vi "Test.vi"() -> ()   [LabVIEW 2022 SP3, in "ZKTimingControl.lvlib" / "TimingControl.lvclass"]
uses:
  TimingControl.lvclass
panel:
  in  "仪器状态":bool
  out "数据":cluster{"启动":bool, "控制命令":T1, "测量参数":T2}={"启动"=FALSE, "控制命令"=enum."加标回收（启动采配水）", "测量参数"={"氨氮"=TRUE, "总磷"=TRUE, "总氮"=TRUE, "CODMn"=TRUE, "CODCr"=FALSE, "氟化物"=FALSE, "挥发酚"=FALSE}}
  in  "布尔":bool
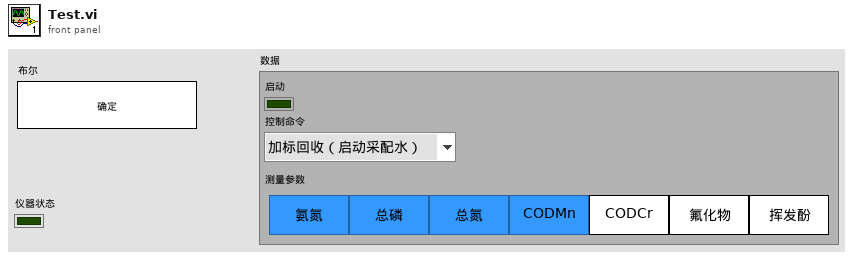
[diagram p1: front panel]
types:
  T1 = typedef "ZKTimingControl.lvlib/TimingControl.lvclass/国标控制命令.ctl" = enum16{"加标回收（启动采配水）", "加标回收（不启动采配水）", "水样测试（启动采配水）", "水样测试（不启动采配水）", "平行样测试（启动采配水）", "平行样测试（不启动采配水）", "集成干预测试"}
  T2 = typedef "ZKTimingControl.lvlib/TimingControl.lvclass/测量参数.ctl" = cluster{"氨氮":bool, "总磷":bool, "总氮":bool, "CODMn":bool, "CODCr":bool, "氟化物":bool, "挥发酚":bool}
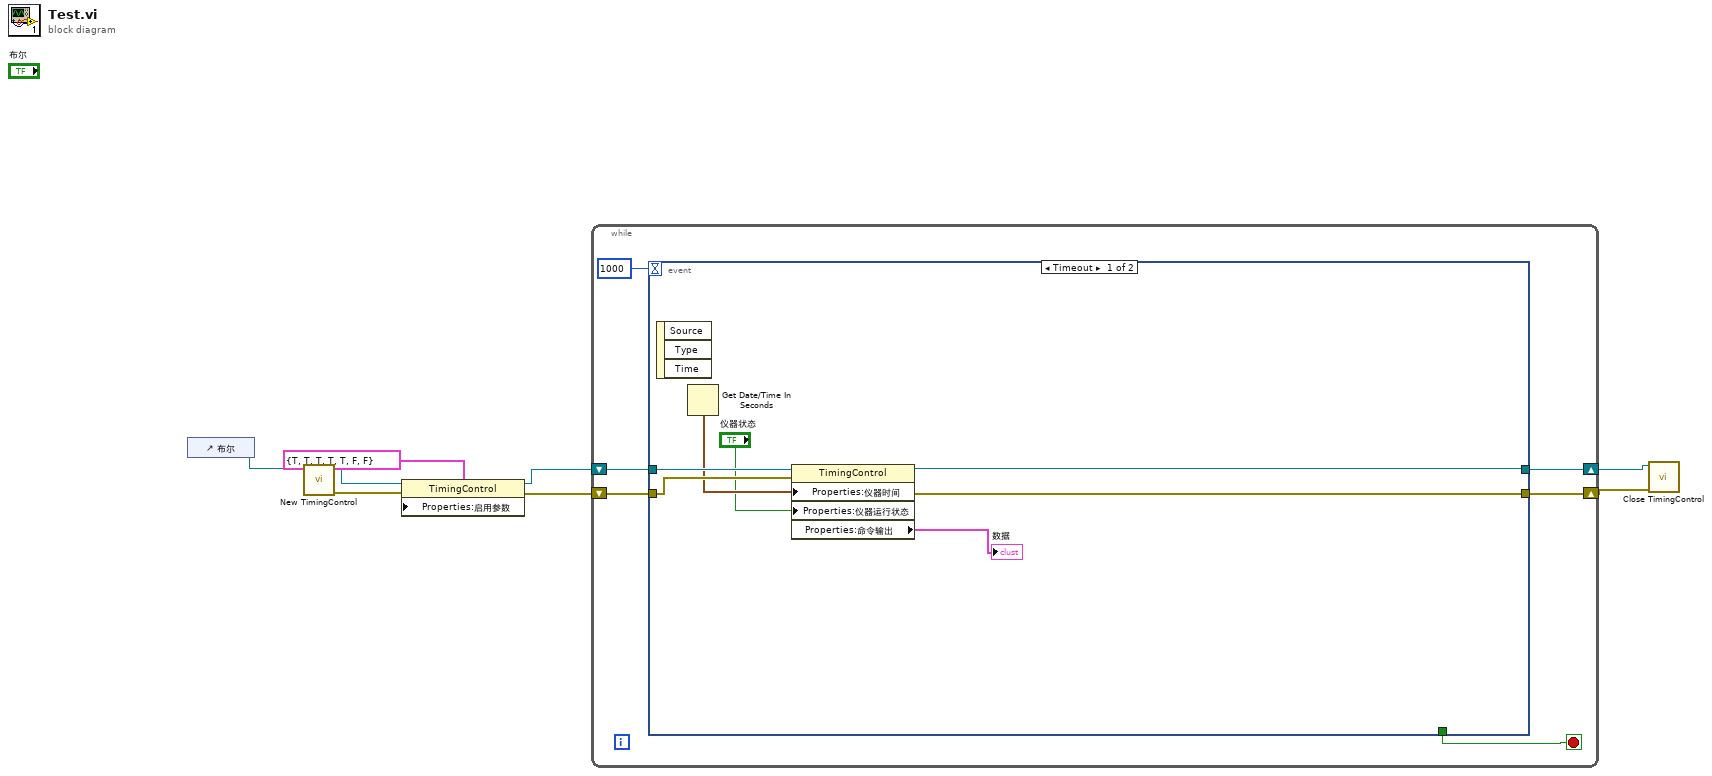
[diagram p0: block diagram]
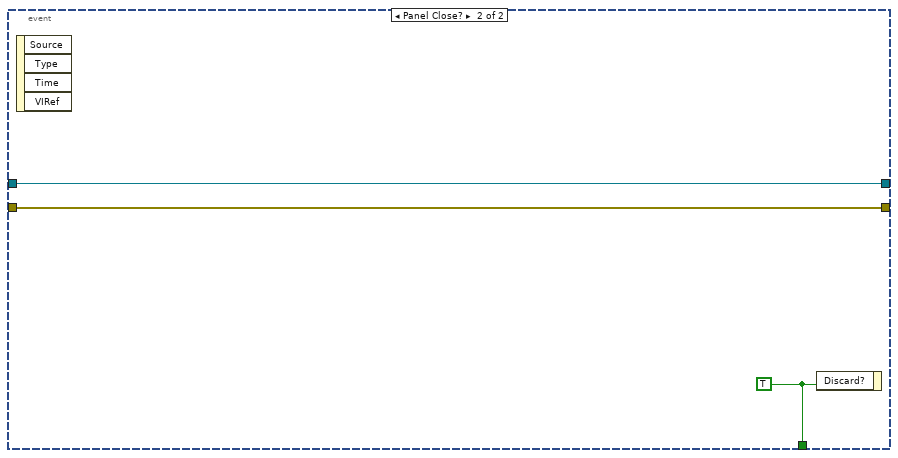
[diagram p2: hidden frame]
diagram:
  n1 = control-ref of="布尔"() -> (w8:refnum<vi>)
  n2 = call "New TimingControl.vi"("Reference"=w8) -> ("error out"=w7:errorcluster, "TimingControl out"=w3:refnum<class "TimingControl.lvclass">)  [unwired: 9 in]
  n3 = property class="TimingControl"(reference=w3, error in=w7, "Properties:启用参数"=T2 {"氨氮"=TRUE, "总磷"=TRUE, "总氮"=TRUE, "CODMn"=TRUE, "CODCr"=TRUE, "氟化物"=FALSE, "挥发酚"=FALSE} ("启用参数")) -> (reference out=w2:refnum<class "TimingControl.lvclass">, error out=w4:errorcluster)
  n4 = while {
    shift-right: [w11] -> w6
    shift-left: w2 -> [w13]
    shift-right: [w10] -> w5
    shift-left: w4 -> [w12]
    stop <- w14 stop-if-true
    n5 = event shown="[0] Timeout" {
      selector: _ -> [_ _]
      dyn-events: _ -> [_ _]
      timeout: 1000 -> [_ _]
      tunnel: [_ w24] -> w14
      tunnel: w13 -> [w18 w23]
      tunnel: w12 -> [w19 w22]
      tunnel: [w21 w23] -> w11
      tunnel: [w20 w22] -> w10
      event Timeout {
        n6 = event-data() -> ()  [unwired: 1 in, 3 out]
        n7 = Get Date/Time In Seconds() -> (seconds since 1Jan1904=w17:timestamp)
        n8 = property class="TimingControl"(reference=w18, error in=w19, "Properties:仪器时间"=w17, "Properties:仪器运行状态"="仪器状态") -> (reference out=w21:refnum<class "TimingControl.lvclass">, error out=w20:errorcluster, "Properties:命令输出"=→"数据":cluster{"启动":bool, "控制命令":T1, "测量参数":T2})
      }
      event Panel Close? {
        w24 = TRUE
        n9 = event-data() -> ()  [unwired: 1 in, 4 out]
        n10 = event-data("Discard?"=w24) -> ()  [unwired: 1 in, 1 out]
      }
    }
  }
  n11 = call "Close TimingControl.vi"("error in (no error)"=w5, "TimingControl in"=w6) -> ()  [unwired: 9 in, 1 out]
